vi "Serial.vi"(8 "error in (no error)":errorcluster, 9 "Clear Log":bool, 10 "write buffer":string="UA[3]\r\n", 11 "VISA resource name":refnum<visa-resource-name>="COM6") -> (0 "error out":errorcluster, 2 "read buffer":string)   [LabVIEW 2017]
uses:
  <vilib>/Instr/_visa.llb/VISA Configure Serial Port (Instr).vi
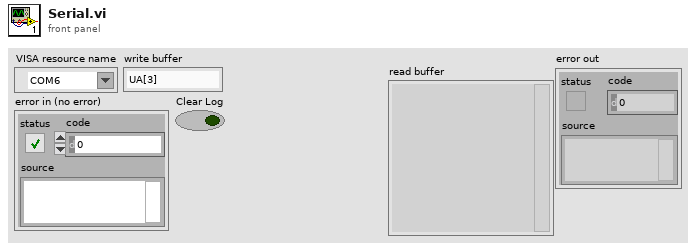
[diagram p1: front panel]
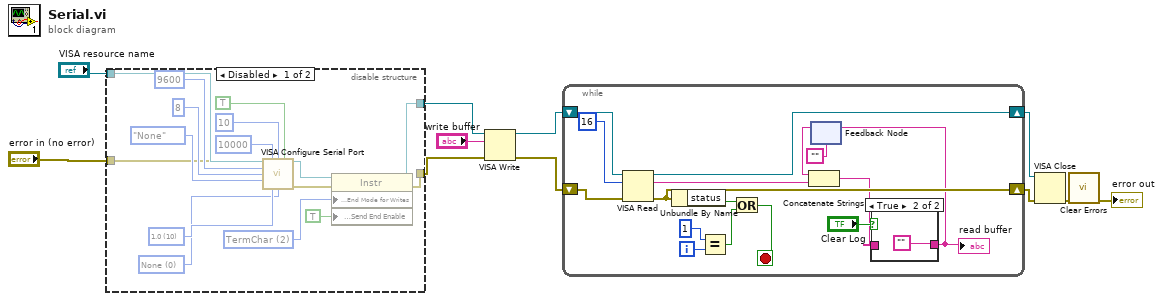
[diagram p0: block diagram]
diagram:
  n1 = disable-structure shown="Disabled" {
    disable-tunnel: "VISA resource name" -> [w27 w29]
    disable-tunnel: "error in (no error)" -> [w21 w28]
    disable-tunnel: [w16 w29] -> w3
    disable-tunnel: [w15 w28] -> w5
    frame Disabled {
      w13 = u16 2 items=["None", "LastBit", "TermChar", "Break"] ("Serial Settings:Serial End Mode for Writes")
      w19 = u16 0 items=["None", "XON/XOFF", "RTS/CTS", "XON/XOFF & RTS/CTS", "DTR/DSR", "XON/XOFF & DTR/DSR"] ("flow control (0:none)")
      w20 = u16 10 items=["1.0"=10, "1.5"=15, "2.0"=20] ("stop bits (10: 1 bit)")
      n2 = call-poly "VISA Configure Serial Port"("VISA resource name"=w27, "timeout (10sec)"=u32 10000, "termination char\n(0xA = '\\n' = LF)"=u8 10 ("termination char\n(0xA = '\\n' = LF)"), "Enable Termination\nChar (T)"=TRUE ("Enable Termination\nChar (T)"), "baud rate (9600)"=u32 9600, "data bits (8)"=u16 8, "parity (0:none)"=enum16{"None", "Odd", "Even", "Mark", "Space"}."None", "error in (no error)"=w21, "stop bits (10: 1 bit)"=w20, "flow control (0:none)"=w19) -> ("VISA resource name out"=w17:refnum<visa-resource-name>, "error out"=w18:errorcluster)  [unwired: 4 in]
      n3 = property class="Instr"(reference=w17, error in=w18, "Serial Settings:End Mode for Writes"=w13, "Message Based Settings:Send End Enable"=TRUE) -> (reference out=w16:refnum<visa-resource-name>, error out=w15:errorcluster)
    }
    frame Enabled {
    }
  }
  n4 = VISA Write(VISA resource name=w3, write buffer="write buffer", error in (no error)=w5) -> (VISA resource name out=w2:refnum<visa-resource-name>, error out=w1:errorcluster)  [unwired: 1 out]
  n5 = while {
    shift-right: [w45] -> w9
    shift-left: w2 -> [w36]
    shift-right: [w40] -> w10
    shift-left: w1 -> [w35]
    i -> [w43]
    stop <- w38 stop-if-true
    n6 = VISA Read(VISA resource name=w36, byte count=u32 16, error in (no error)=w35) -> (VISA resource name out=w45:refnum<visa-resource-name>, read buffer=w44:string, error out=w40:errorcluster)  [unwired: 1 out]
    n7 = Unbundle By Name(w40) -> ("status"=w37:bool)
    n8 = Equal?(x=1, y=w43) -> (x = y?=w39:bool)
    n9 = Or(x=w37, y=w39) -> (x .or. y?=w38:bool)
    n10 = feedback #1("") -> (w34:string)
    n11 = Concatenate Strings(w34, w44) -> (w31:string)
    n12 = case shown="True" "Clear Log" {
      tunnel: w31 -> [w46 _]
      tunnel: [w46 ""] -> w30
      frame False {
      }
      frame True {
      }
    }
    "read buffer" <- w30
    n13 = feedback-in #1(w30) -> ()
  }
  n14 = VISA Close(VISA resource name=w9, error in (no error)=w10) -> (error out=w7:errorcluster)
  n15 = call <vilib>:"Clear Errors.vi"("error in (no error)"=w7) -> ("error out"=→"error out":errorcluster)  [unwired: 5 in, 1 out]
